vi "ABB Get norma 5000 rdgs.vi"(4 "Rated":T1, 6 "Simulation rdgs":cluster{"V":dbl, "A":dbl, "pwr factor":dbl} {"pwr factor" scale=0.0..1.0; "A" scale=0.0..100.0; "V" scale=0.0..10000.0}, 7 "simulate":bool, 8 "norma 5000 parms in":T4, 9 "Simulate Mode":T2(ring)) -> (0 "norma 5000 parms out":T4, 1 "L 3":T3, 2 "L 2":T3, 3 "L1":T3, 5 "Total":T3)   [LabVIEW 2017]
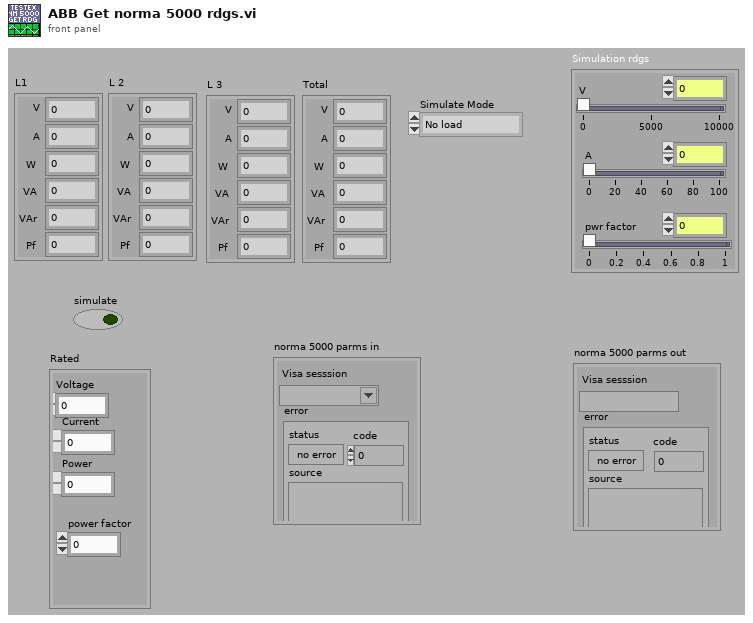
[diagram p1: front panel]
types:
  T1 = cluster{"Voltage":dbl, "Current":dbl, "Power":dbl, "power factor":dbl}
  T2 = enum16{"No load", "Locked Rotor", "Heat run", "NoLd heat run", "Partial heat run"}
  T3 = cluster{"V":dbl, "A":dbl, "W":dbl, "VA":dbl, "VAr":dbl, "Pf":dbl}
  T4 = cluster{"Visa sesssion":refnum<visa-resource-name>, "error":errorcluster}
  T5 = cluster{"[0]":dbl, "[1]":dbl, "[2]":dbl, "[3]":dbl, "[4]":dbl, "[5]":dbl}
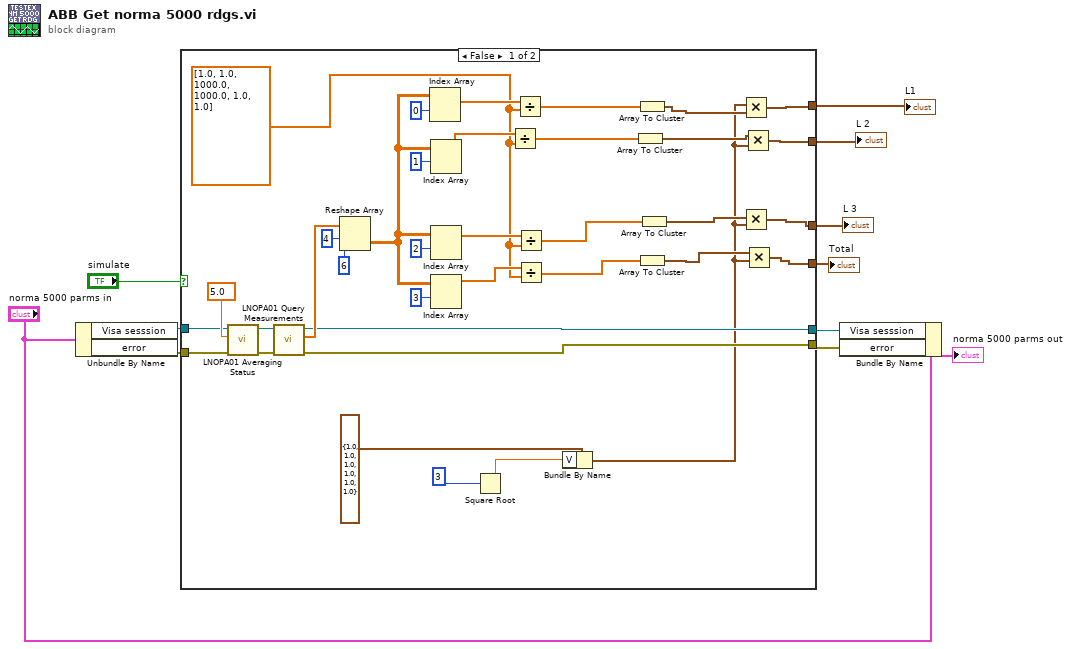
[diagram p0: block diagram]
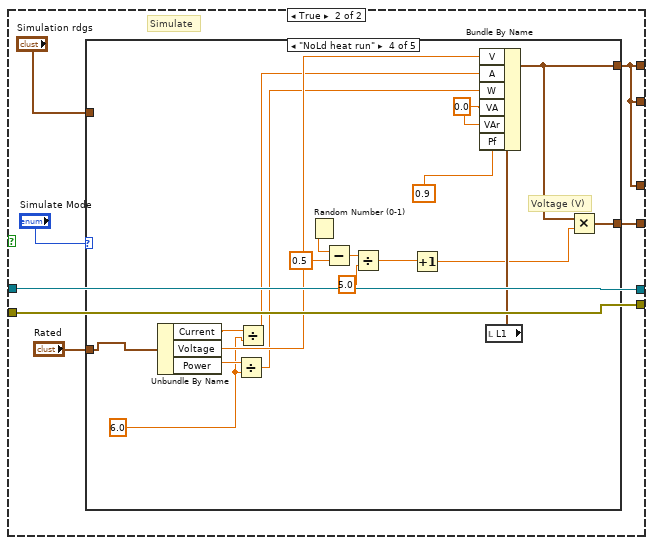
[diagram p2: hidden frame]
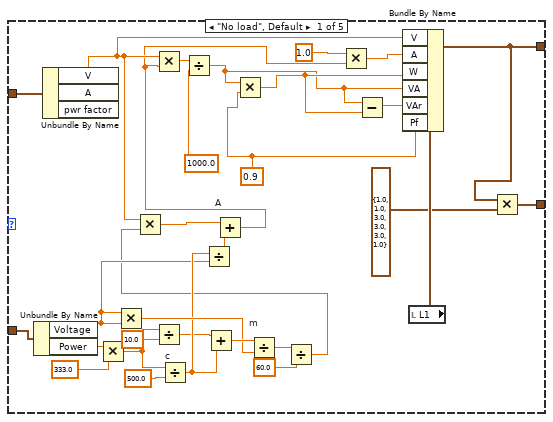
[diagram p3: hidden frame]
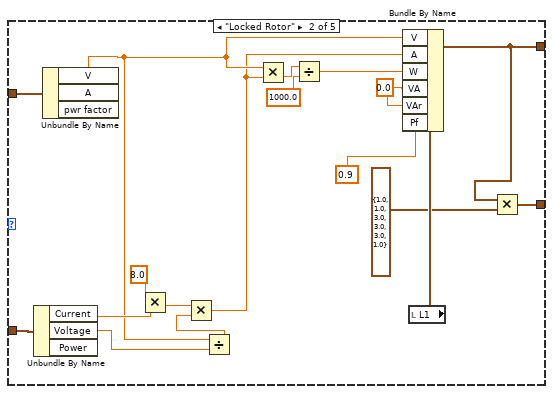
[diagram p4: hidden frame]
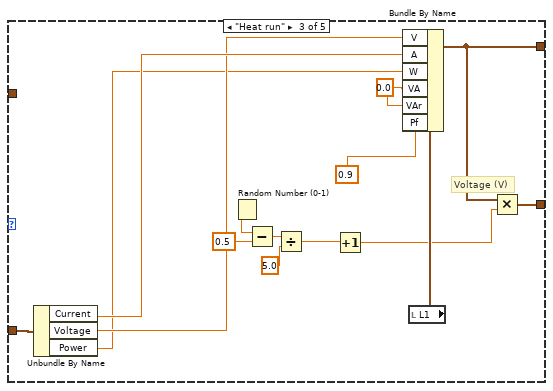
[diagram p5: hidden frame]
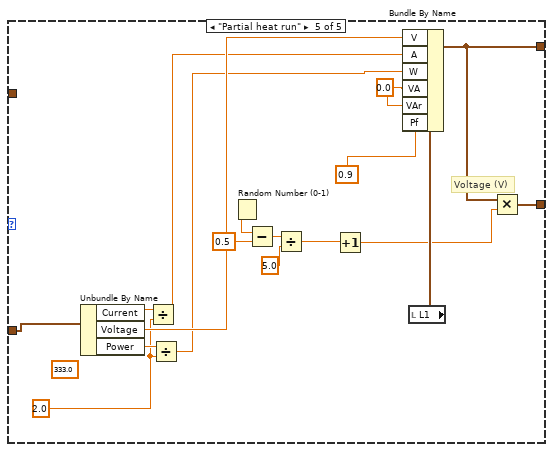
[diagram p6: hidden frame]
diagram:
  n1 = Unbundle By Name("norma 5000 parms in") -> ("Visa sesssion"=w10:refnum<visa-resource-name>, "error"=w9:errorcluster)
  n2 = case shown="False" "simulate" {
    tunnel: w9 -> [w36 w53]
    tunnel: w10 -> [w35 w54]
    tunnel: [w34 w54] -> w7
    tunnel: [w33 w53] -> w6
    tunnel: [w20 w51] -> w4
    tunnel: [w18 w51] -> w1
    tunnel: [w16 w51] -> w2
    tunnel: [w14 w50] -> w3
    frame False {
      w25 = dbl[] [1.0, 1.0, 1000.0, 1000.0, 1.0, 1.0]
      n3 = call "LNOPA01 Averaging Status.vi"("error in (no error)"=w36, "Timeout"=5.0, "VISA session"=w35) -> ("error out"=w39:errorcluster, "dup VISA session"=w38:refnum<visa-resource-name>)  [unwired: 6 in, 1 out]
      n4 = call "LNOPA01 Query Measurements.vi"("error in (no error)"=w39, "VISA session"=w38) -> ("error out"=w33:errorcluster, "Data"=w47:dbl[], "dup VISA session"=w34:refnum<visa-resource-name>)  [unwired: 7 in]
      n5 = Reshape Array(w47, 4 ("Dimension Size"), 6 ("Dimension Size")) -> (w37:dbl[][])
      n6 = Index Array(array=w37, index (row)=0 ("Index")) -> (element=w31:dbl[])  [unwired: 1 in]
      n7 = Index Array(array=w37, index (row)=1 ("Index")) -> (element=w29:dbl[])  [unwired: 1 in]
      n8 = Index Array(array=w37, index (row)=2 ("Index")) -> (element=w27:dbl[])  [unwired: 1 in]
      n9 = Index Array(array=w37, index (row)=3 ("Index")) -> (element=w26:dbl[])  [unwired: 1 in]
      n10 = Square Root(x=3) -> (sqrt(x)=w13:dbl)
      n11 = Divide(x=w29, y=w25) -> (x/y=w30:dbl[])
      n12 = Divide(x=w31, y=w25) -> (x/y=w32:dbl[])
      n13 = Divide(x=w27, y=w25) -> (x/y=w28:dbl[])
      n14 = Divide(x=w26, y=w25) -> (x/y=w24:dbl[])
      n15 = Bundle By Name(cluster=T3 {"V"=1.0, "A"=1.0, "W"=1.0, "VA"=1.0, "VAr"=1.0, "Pf"=1.0} ("L1"), "V"=w13) -> (w12:T3)
      n16 = Array To Cluster(array=w30) -> (cluster=w19:T5)
      n17 = Array To Cluster(array=w32) -> (cluster=w21:T5)
      n18 = Array To Cluster(array=w24) -> (cluster=w15:T5)
      n19 = Array To Cluster(array=w28) -> (cluster=w17:T5)
      n20 = Multiply(x=w12, y=w21) -> (x*y=w20:cluster{dbl, dbl, dbl, dbl, dbl, dbl})
      n21 = Multiply(x=w17, y=w12) -> (x*y=w16:cluster{dbl, dbl, dbl, dbl, dbl, dbl})
      n22 = Multiply(x=w19, y=w12) -> (x*y=w18:cluster{dbl, dbl, dbl, dbl, dbl, dbl})
      n23 = Multiply(x=w15, y=w12) -> (x*y=w14:cluster{dbl, dbl, dbl, dbl, dbl, dbl})
    }
    frame True {
      # "Simulate"
      n24 = case shown="\"NoLd heat run\"" "Simulate Mode" {
        tunnel: "Simulation rdgs" -> [w85 w103 _ _ _]
        tunnel: [w81 w101 w104 w124 w141] -> w51
        tunnel: [w79 w99 w117 w135 w153] -> w50
        tunnel: "Rated" -> [w75 w98 w116 w123 w140]
        frame "No load", Default {
          w64 = 0.9
          n25 = Unbundle By Name(w75) -> ("Voltage"=w66:dbl, "Power"=w74:dbl)
          n26 = Unbundle By Name(w85) -> ("V"=w69:dbl)  [unwired: 2 out]
          n27 = Multiply(x=w74, y=333.0) -> (x*y=w62:dbl)
          n28 = Multiply(x=w66, y=w66) -> (x*y=w70:dbl)
          n29 = Divide(x=w62, y=10.0) -> (x/y=w60:dbl)
          n30 = Divide "c"(x=w62, y=500.0) -> (x/y=w67:dbl)
          n31 = Divide(x=w67, y=w66) -> (x/y=w65:dbl)
          n32 = Add(x=w60, y=w67) -> (x+y=w71:dbl)
          n33 = Divide "m"(x=w71, y=w70) -> (x/y=w59:dbl)
          n34 = Divide(x=w59, y=60.0) -> (x/y=w57:dbl)
          n35 = Multiply(x=w69, y=w57) -> (x*y=w68:dbl)
          n36 = Add "A"(x=w68, y=w65) -> (x+y=w63:dbl)
          n37 = Multiply(x=w69, y=w63) -> (x*y=w77:dbl)
          n38 = Divide(x=w77, y=1000.0) -> (x/y=w78:dbl)
          n39 = Multiply(x=w78, y=w64) -> (x*y=w83:dbl)
          n40 = Multiply(x=1.0, y=w63) -> (x*y=w56:dbl)
          n41 = Subtract(x=w78, y=w83) -> (x-y=w82:dbl)
          n42 = local read "L1"() -> (w84:T3)
          n43 = Bundle By Name(cluster=w84, "V"=w69, "A"=w56, "W"=w83, "VA"=w78, "VAr"=w82, "Pf"=w64) -> (w81:T3)
          n44 = Multiply(x=w81, y=T3 {"V"=1.0, "A"=1.0, "W"=3.0, "VA"=3.0, "VAr"=3.0, "Pf"=1.0} ("L1")) -> (x*y=w79:T3)
        }
        frame "Locked Rotor" {
          w89 = 0.0 ("VA")
          n45 = Unbundle By Name(w98) -> ("Current"=w96:dbl, "Voltage"=w94:dbl)  [unwired: 1 out]
          n46 = Unbundle By Name(w103) -> ("V"=w91:dbl)  [unwired: 2 out]
          n47 = Multiply(x=8.0, y=w96) -> (x*y=w92:dbl)
          n48 = Divide(x=w91, y=w94) -> (x/y=w93:dbl)
          n49 = Multiply(x=w92, y=w93) -> (x*y=w90:dbl)
          n50 = Multiply(x=w91, y=w90) -> (x*y=w87:dbl)
          n51 = Divide(x=w87, y=1000.0) -> (x/y=w88:dbl)
          n52 = local read "L1"() -> (w102:T3)
          n53 = Bundle By Name(cluster=w102, "V"=w91, "A"=w90, "W"=w88, "VA"=w89, "VAr"=w89, "Pf"=0.9) -> (w101:T3)
          n54 = Multiply(x=w101, y=T3 {"V"=1.0, "A"=1.0, "W"=3.0, "VA"=3.0, "VAr"=3.0, "Pf"=1.0} ("L1")) -> (x*y=w99:T3)
        }
        frame "Heat run" {
          w114 = 0.0 ("VA")
          # "Voltage (V)"
          n55 = Unbundle By Name(w116) -> ("Current"=w113:dbl, "Voltage"=w112:dbl, "Power"=w111:dbl)
          n56 = Random Number (0-1)() -> (number: 0 to 1=w109:dbl)
          n57 = Subtract(x=w109, y=0.5) -> (x-y=w107:dbl)
          n58 = Divide(x=w107, y=5.0) -> (x/y=w106:dbl)
          n59 = Increment(x=w106) -> (x+1=w105:dbl)
          n60 = local read "L1"() -> (w118:T3)
          n61 = Bundle By Name(cluster=w118, "V"=w112, "A"=w113, "W"=w111, "VA"=w114, "VAr"=w114, "Pf"=0.9) -> (w104:T3)
          n62 = Multiply(x=w104, y=w105) -> (x*y=w117:T3)
        }
        frame "NoLd heat run" {
          w119 = 6.0 ("Voltage")
          w133 = 0.0 ("VA")
          # "Voltage (V)"
          n63 = Unbundle By Name(w123) -> ("Current"=w132:dbl, "Voltage"=w131:dbl, "Power"=w120:dbl)
          n64 = Divide(x=w120, y=w119) -> (x/y=w121:dbl)
          n65 = Divide(x=w132, y=w119) -> (x/y=w122:dbl)
          n66 = Random Number (0-1)() -> (number: 0 to 1=w129:dbl)
          n67 = Subtract(x=w129, y=0.5) -> (x-y=w127:dbl)
          n68 = Divide(x=w127, y=5.0) -> (x/y=w126:dbl)
          n69 = Increment(x=w126) -> (x+1=w125:dbl)
          n70 = local read "L1"() -> (w136:T3)
          n71 = Bundle By Name(cluster=w136, "V"=w131, "A"=w122, "W"=w121, "VA"=w133, "VAr"=w133, "Pf"=0.9) -> (w124:T3)
          n72 = Multiply(x=w124, y=w125) -> (x*y=w135:T3)
        }
        frame "Partial heat run" {
          w137 = 2.0 ("Voltage")
          w151 = 0.0 ("VA")
          (unwired) 333.0 ("y")
          # "Voltage (V)"
          n73 = Unbundle By Name(w140) -> ("Current"=w150:dbl, "Voltage"=w149:dbl, "Power"=w148:dbl)
          n74 = Divide(x=w150, y=w137) -> (x/y=w139:dbl)
          n75 = Divide(x=w148, y=w137) -> (x/y=w138:dbl)
          n76 = Random Number (0-1)() -> (number: 0 to 1=w146:dbl)
          n77 = Subtract(x=w146, y=0.5) -> (x-y=w144:dbl)
          n78 = Divide(x=w144, y=5.0) -> (x/y=w143:dbl)
          n79 = Increment(x=w143) -> (x+1=w142:dbl)
          n80 = local read "L1"() -> (w154:T3)
          n81 = Bundle By Name(cluster=w154, "V"=w149, "A"=w139, "W"=w138, "VA"=w151, "VAr"=w151, "Pf"=0.9) -> (w141:T3)
          n82 = Multiply(x=w141, y=w142) -> (x*y=w153:T3)
        }
      }
    }
  }
  "L1" <- w4
  "L 2" <- w1
  "L 3" <- w2
  "Total" <- w3
  n83 = Bundle By Name(cluster="norma 5000 parms in", "Visa sesssion"=w7, "error"=w6) -> (→"norma 5000 parms out":T4)
